vi "SPC_write_data_block.vi"(4 "Data Buffer":u16[](array[numeric]), 5 "Block":i32 min=0 max=65535 step=1, 6 "Page":i32 min=0 max=65535 step=1, 7 "Module No":i16 min=0 max=7 step=1, 8 "Error In":errorcluster, 9 "To":i16=64 min=0 max=4095 step=1, 10 "From":i16 min=0 max=4095 step=1, 11 "DLL Path":path) -> (0 "Error Out":errorcluster, 2 "Module No":i16 min=0 max=7 step=1, 3 "DLL Path":path)   [LabVIEW 2017]
doc: "The procedure reads data from the buffer ‘data’ in the PC and writes it to a block of the memory defined by the parameters ‘block’ and ‘page’ on the SPC module ‘mod_no’. The procedure is used to write data from the from PC memory to the memory of the SPC module. \n\nParameters ‘from’ and ‘to’ define the address range inside the buffer ‘data’ and the address range inside the SPC memory block to which the data will be written. The range of the parameters ‘block’ and ‘page’ depends on the actual configuration of the SPC memory (see SPC_configure_memory). \n\nThe assumption is done that frames_per_page is equal 1 ( page = frame ) (see 'Memory Configuration).\nTo provide correct access to the SPC memory it is required that the function SPC_configure_memory be called ( in normal operation modes) before the first call of SPC_write_data_block. This function also delivers the required information about the block/page structure of the SPC memory.\n\ninfo@becker-hickl.com"
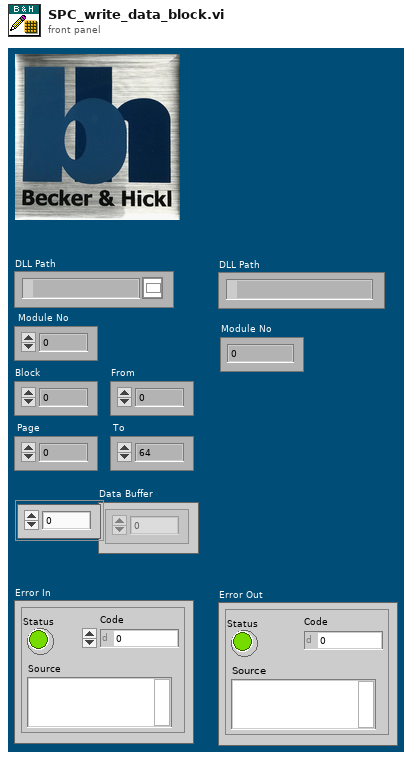
[diagram p1: front panel]
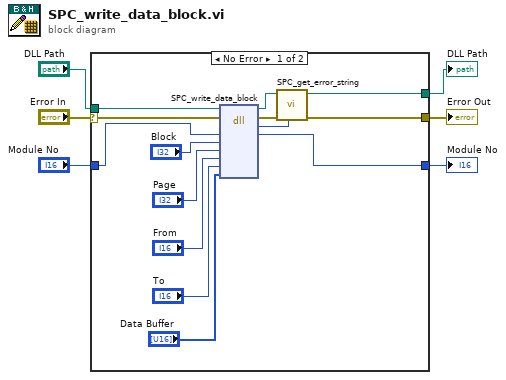
[diagram p0: block diagram]
diagram:
  n1 = case shown="No Error" "Error In" {
    selector: "Error In" -> [w15 w23]
    tunnel: "DLL Path" -> [w16 w22]
    tunnel: [w9 w22] -> w5
    tunnel: [w11 w23] -> w4
    tunnel: "Module No" -> [w14 w21]
    tunnel: [w13 w21] -> w1
    frame No Error {
      n2 = dll-call lib="D:/spcm/lib/lab_view/lv10.0/spcm32.dll" fn="SPC_write_data_block"(path in=w16, error in=w15, "mod_no"=w14, "block"="Block", "page"="Page", "from"="From", "to"="To", "data"="Data Buffer") -> (path out=w10:path, error out=w12:errorcluster, "return type"=w8:i16, "mod_no"=w13:i16)  [unwired: 6 in]
      n3 = call "SPC_get_error_string.vi"("ErrorID"=w8, "Error In"=w12, "DLL Path"=w10) -> ("Error Out"=w11:errorcluster, "DLL Path"=w9:path)  [unwired: 6 in, 1 out]
    }
    frame Error {
    }
  }
  "DLL Path" <- w5
  "Error Out" <- w4
  "Module No" <- w1
